vi "Destroy.vi"(0 "reference in":refnum<class "DCIR_HPPC.lvclass">, 5 "Error In":errorcluster) -> (14 "reference out":refnum<class "DCIR_HPPC.lvclass">, 19 "Error Out":errorcluster)   [LabVIEW 2023, in "DCIR_HPPC.lvclass"]
uses:
  DCIR_HPPC.lvclass
  DCIR_HPPC.lvclass/DCIR_HPPC.ctl
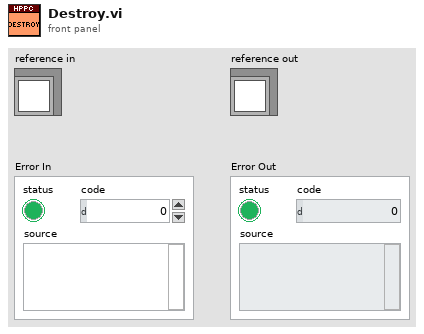
[diagram p1: front panel]
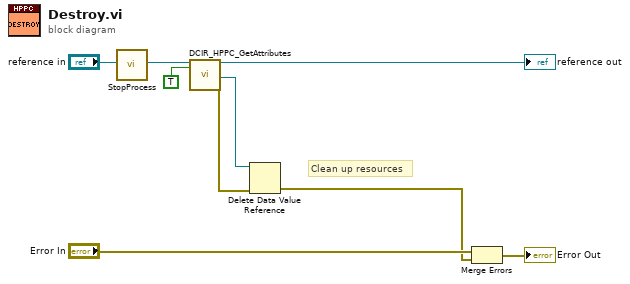
[diagram p0: block diagram]
diagram:
  # "Clean up resources"
  n1 = call "StopProcess.vi"("reference in"="reference in") -> ("reference out"=w2:refnum<class "DCIR_HPPC.lvclass">)  [unwired: 17 in, 1 out]
  n2 = call "DCIR_HPPC_GetAttributes.vi"("reference in"=w2, "OnlyGetDvrReference(False)"=TRUE) -> ("reference out"=→"reference out":refnum<class "DCIR_HPPC.lvclass">, "DataRef"=w1:refnum<data-value>, "Error Out"=w7:errorcluster)  [unwired: 14 in, 1 out]
  n3 = Delete Data Value Reference(data value reference=w1, error in=w7) -> (error out=w5:errorcluster)  [unwired: 1 out]
  n4 = Merge Errors("Error In", w5) -> (→"Error Out":errorcluster)
